vi "Put Helper Loop to Sleep.vi"(8 "error in":errorcluster, 11 "Local Events":T1) -> (0 "error out":errorcluster)   [LabVIEW 2020, in "Lock-in amplifier.lvlib" / "Local Events.lvlib"]
doc: "____\nPantherLAB Templates 1.0.0.5\nCopyright (c) 2022, PantherLAB"
uses:
  Local Events.lvlib
  Local Events--cluster.ctl
  Support/Continuous acq data -- cluster.ctl
  Lock-in amplifier.lvlib
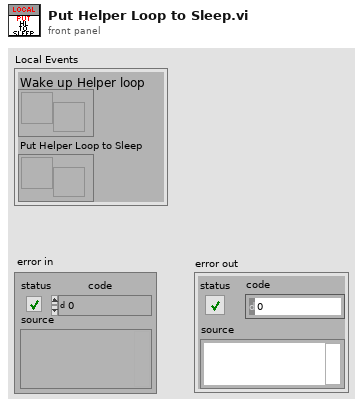
[diagram p1: front panel]
types:
  T1 = typedef "Lock-in amplifier.lvlib/Local Events.lvlib/Local Events--cluster.ctl" = cluster{"Wake up Helper loop":refnum<user-event>, "Put Helper Loop to Sleep":refnum<user-event>}
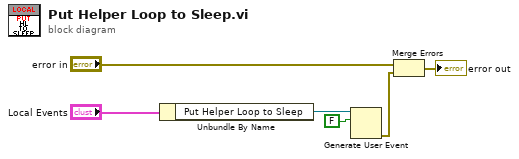
[diagram p0: block diagram]
diagram:
  n1 = Unbundle By Name("Local Events") -> ("Put Helper Loop to Sleep"=w2:refnum<user-event>)
  n2 = Generate User Event(user event=w2, event data cluster=FALSE ("event data")) -> (error out=w5:errorcluster)  [unwired: 2 in, 1 out]
  n3 = Merge Errors("error in", w5) -> (→"error out":errorcluster)
